vi "HDLC Zero Bit Stuffing.vi"(1 "Read Operation (T)":bool, 2 "Data in":bool[](array[boolean])) -> (0 "Data Out":bool[](array[boolean]))   [LabVIEW 2019]
doc: "HDLC protocol Flag has a unique binary pattern and, in order to avoid that the data field to transmit contains the same pattern, \"zero bit insertion\" technique is used.\nThis technique specifies to the transmitting device the insertion of a binary 0 every five consecutive\nbinary \"1\". The receiving device must be have the capability to recognize the zero and to delete\ninto information field every \"0\" followed by consecutive file binary \"1\".\nUSAGE:\nThis VI does both Receiving and transmitting part. Place this VI in transmitting chain after complete message created including all four fields of HDLC and Wire False to \"Read Operation(T)\" button.\nFor Reception After extracting message within flag(by using [HDLC] Flag Check.vi) place this VI and wire True to \"Read Operation(T)\" button."
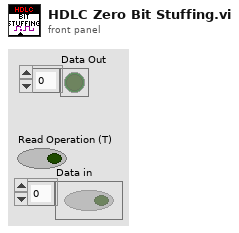
[diagram p1: front panel]
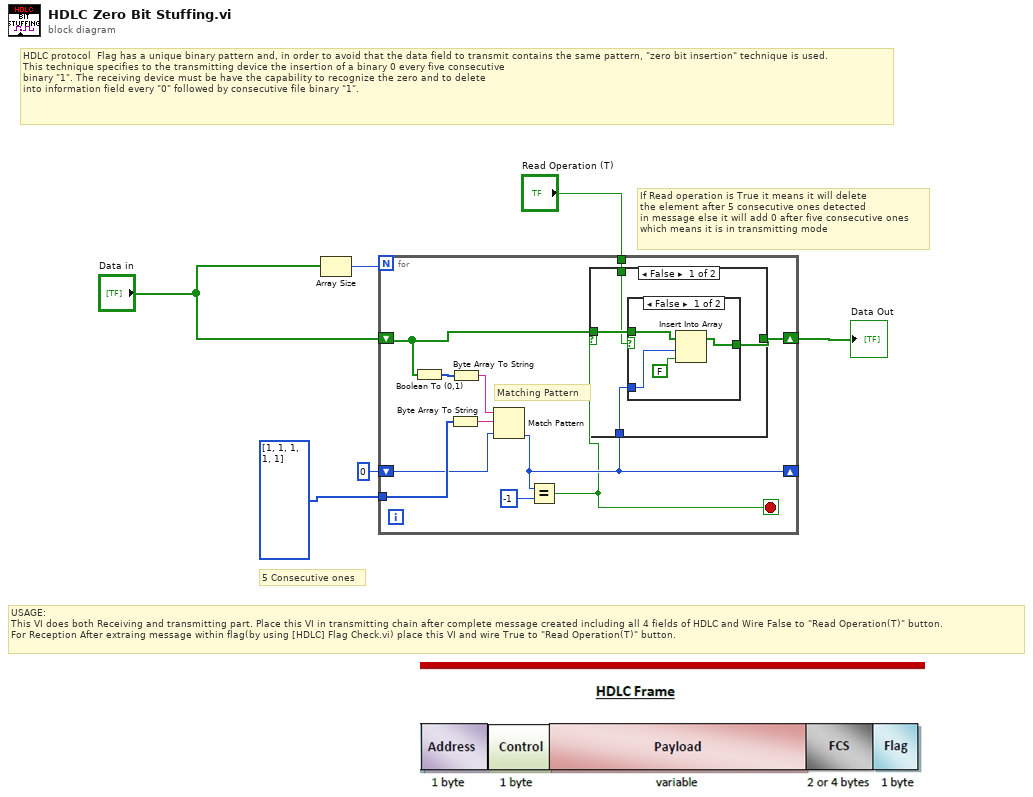
[diagram p0: block diagram]
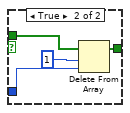
[diagram p2: hidden frame]
diagram:
  # "USAGE:\nThis VI does both Receiving and transmitting part. Place this VI in transmitting chain after complete message created including all 4 fields of HDLC and Wire False to \"Read Operation(T)\" button.\nFor Reception After extraing message within flag(by using [HDLC] Flag Check.vi) place this VI and wire True to \"Read Operation(T)\" button."
  # "HDLC protocol  Flag has a unique binary pattern and, in order to avoid that the data field to transmit contains the same pattern, \"zero bit insertion\" technique is used.\nThis technique specifies to the transmitting device the insertion of a binary 0 every five consecutive\nbinary \"1\". The receiving device must be have the capability to recognize the zero and to delete\ninto information field every \"0\" followed by consecutive file binary \"1\"."
  # "If Read operation is True it means it will delete\nthe element after 5 consecutive ones detected \nin message else it will add 0 after five consecutive ones\nwhich means it is in transmitting mode"
  # "5 Consecutive ones"
  n1 = Array Size(array="Data in") -> (size(s)=w4:i32)
  n2 = for {
    N: w4 -> [_]
    tunnel: i16[] [1, 1, 1, 1, 1] ("subarray") -> [w15]
    shift-right: [w12] -> _
    shift-left: 0 ("offset past match") -> [w13]
    shift-right: [w11] -> w1
    shift-left: "Data in" -> [w9]
    tunnel: "Read Operation (T)" -> [w8]
    stop <- w10 stop-if-true
    # "Matching Pattern"
    n3 = Boolean To (0,1)(Boolean=w9) -> (0, 1=w7:i16[])
    n4 = Byte Array To String(unsigned byte array=w15) -> (string=w16:string)
    n5 = Byte Array To String(unsigned byte array=w7) -> (string=w17:string)
    n6 = Match Pattern(string=w17, regular expression=w16, offset (0)=w13) -> (offset past match=w12:i32)  [unwired: 3 out]
    n7 = Equal?(x=w12, y=-1) -> (x = y?=w10:bool)
    n8 = case shown="False" w10 {
      tunnel: w9 -> [w21 w30]
      tunnel: w12 -> [w20 _]
      tunnel: [w19 w30] -> w11
      tunnel: w8 -> [w18 _]
      frame False {
        n9 = case shown="False" w18 {
          tunnel: w21 -> [w25 w29]
          tunnel: w20 -> [w24 w28]
          tunnel: [w23 w26] -> w19
          frame False {
            n10 = Insert Into Array(array=w25, index=w24, new element=FALSE ("new element/subarray")) -> (w23:bool[])
          }
          frame True {
            n11 = Delete From Array(array=w29, length=1, index=w28) -> (array with subset deleted=w26:bool[])  [unwired: 1 out]
          }
        }
      }
      frame True {
      }
    }
  }
  "Data Out" <- w1
